vi "Noise Gate.vi"(1 "Gate Value":dbl, 2 "Value In":dbl) -> (6 "Value Out":dbl)   [LabVIEW 2012]
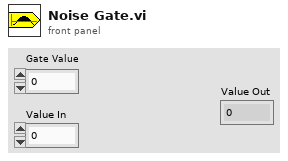
[diagram p1: front panel]
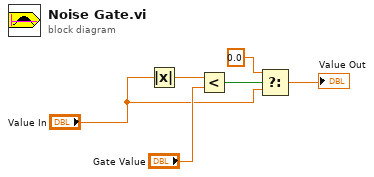
[diagram p0: block diagram]
diagram:
  n1 = Absolute Value(x="Value In") -> (abs(x)=w6:dbl)
  n2 = Less?(x=w6, y="Gate Value") -> (x < y?=w5:bool)
  n3 = Select(t=0.0, s=w5, f="Value In") -> (s? t:f=→"Value Out":dbl)
